vi "HdrDataWrite.vi"(8 "error in (no error)":errorcluster, 11 "Interface.lvclass":refnum<class "Interface.lvclass">) -> (0 "error out":errorcluster, 3 "Interface.lvclassOut":refnum<class "Interface.lvclass">)   [LabVIEW 2019, in "Interface.lvclass"]
doc: "Ce VI sauvegarde les données d'acquisition pour en garder une copie de sécurité qui peut être rappeller en cas de panne."
uses:
  Interface.lvclass
  ScanParams.ctl
  Interface.lvclass/Interface.ctl
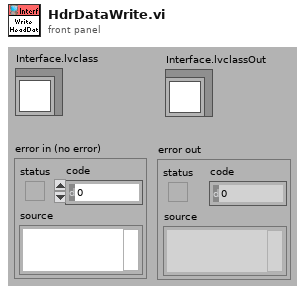
[diagram p1: front panel]
types:
  T1 = typedef "Interface.lvclass/ScanParams.ctl" = cluster{"Entête":string, "Scan list":string[], "NbCourbe":i32, "IndCourbe":i64, "NomDon":string[], "Session ":i32, "Date":string, "Time":string, "VarParams":string[][], "UserName":string, "ScanTableSize":i32[], "VarPar list":string[]}
  T2 = enum16{"open", "replace", "create", "open or create", "replace or create", "replace or create with confirmation"}
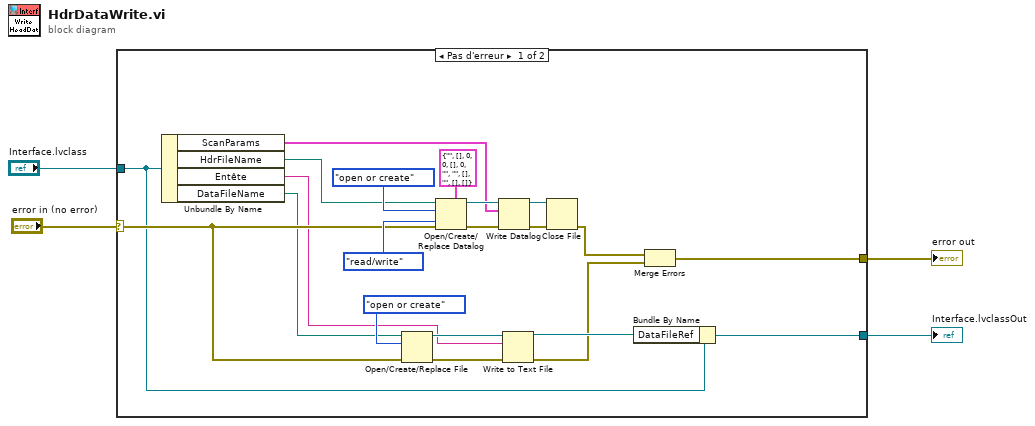
[diagram p0: block diagram]
diagram:
  n1 = case shown="Pas d'erreur" "error in (no error)" {
    selector: "error in (no error)" -> [w14 w27]
    tunnel: [w7 w27] -> w3
    tunnel: "Interface.lvclass" -> [w12 w26]
    tunnel: [w10 w26] -> w1
    frame No Error {
      n2 = Unbundle By Name(w12) -> ("ScanParams"=w18:T1, "HdrFileName"=w19:path, "Entête"=w13:string, "DataFileName"=w6:path)
      n3 = Open/Create/Replace File(file path (use dialog)=w6, error in=w14, operation (0:open)=T2."open or create" ("opération (0 : open)")) -> (refnum out=w16:refnum<file>, error out=w17:errorcluster)  [unwired: 3 in, 1 out]
      n4 = Open/Create/Replace Datalog(5:T1 {"Entête"="", "Scan list"=[], "NbCourbe"=0, "IndCourbe"=0, "NomDon"=[], "Session "=0, "Date"="", "Time"="", "VarParams"=[], "UserName"="", "ScanTableSize"=[], "VarPar list"=[]} ("HdrSaf"), 8:w14, 9:enum16{"read/write", "read-only", "write-only"}."read/write" ("accès (0 : read/write)"), 10:T2."open or create" ("opération (0 : open)"), 11:w19) -> (0:w24:errorcluster, 3:w25:refnum<k1>)  [unwired: 1 in, 1 out]
      n5 = Write Datalog(4:w24, 6:w18, 7:w25) -> (0:w22:errorcluster, 3:w23:refnum<k1>)
      n6 = Write to Text File(file (use dialog)=w16, text=w13, error in=w17) -> (refnum out=w11:refnum<file>, error out=w8:errorcluster)  [unwired: 1 in, 1 out]
      n7 = Close File(refnum=w23, error in=w22) -> (error out=w9:errorcluster)  [unwired: 1 out]
      n8 = Bundle By Name(cluster=w12, "DataFileRef"=w11) -> (w10:refnum<class "Interface.lvclass">)
      n9 = Merge Errors(w9, w8) -> (w7:errorcluster)
    }
    frame Error {
    }
  }
  "error out" <- w3
  "Interface.lvclassOut" <- w1
